vi "BuildSysexMsgCapabilityQuery.vi"(8 "error in":errorcluster) -> (0 "error out":errorcluster, 2 "GetCapabilitiesMessage":u8[](array[numeric]) format="%x", 4 "ReplyFirstByte":T1=224 items=["ANALOG_IO_MESSAGE"=224, "DIGITAL_IO_MESSAGE"=144, "REPORT_ANALOG_PIN"=192, "REPORT_DIGITAL_PORT"=208, "START_SYSEX"=240, "END_SYSEX"=247, "SET_PIN_MODE"=244, "SET_DIGITAL_PIN_VALUE"=245, "PROTOCOL_VERSION"=249, "SYSTEM_RESET"=255, "SYSEX.EXTENDED_ID"=0, "SYSEX.RESERVED_USER_COMMANDs"=1, "SYSEX.ANALOG_MAPPING_QUERY"=105, "SYSEX.ANALOG_MAPPING_RESPONSE"=106, "SYSEX.CAPABILITY_QUERY"=107, "SYSEX.CAPABILITY_RESPONSE"=108, "SYSEX.PIN_STATE_QUERY"=109, "SYSEX.PIN_STATE_RESPONSE"=110, "SYSEX.REPORT_FIRMWARE"=121, "SYSEX.EXTENDED_ANALOG"=111, "SYSEX.STRING_DATA"=113, "SYSEX.REALTIME"=127, "SYSEX.NON_REALTIME"=126, "SYSEX.SAMPLING_INTERVAL"=122, "FEATURES.SYSEX.I2C_READ_WRITE"=118, "FEATURES.SYSEX.I2C_REPLY"=119, "FEATURES.SYSEX.I2C_CONFIG"=120], 6 "ReplyLength":i32=-1)   [LabVIEW 2020, in "FirmataClient.lvlib"]
doc: "Builds the message according to the Firmata Protocol Requirements. \n- https://github.com/firmata/protocol\n- https://github.com/firmata/protocol/blob/master/protocol.md"
uses:
  Controls/FirmataProtocolConstants.ctl
  FirmataClient.lvlib
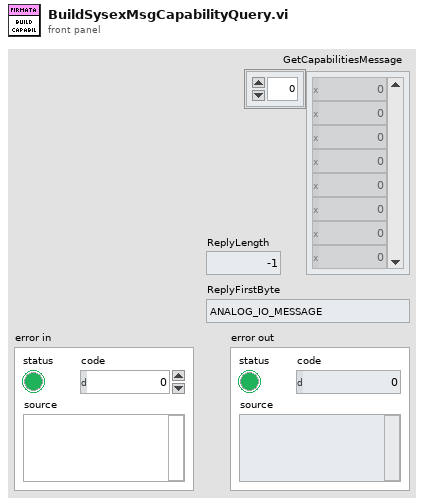
[diagram p1: front panel]
types:
  T1 = typedef "FirmataClient.lvlib/FirmataProtocolConstants.ctl" = u16
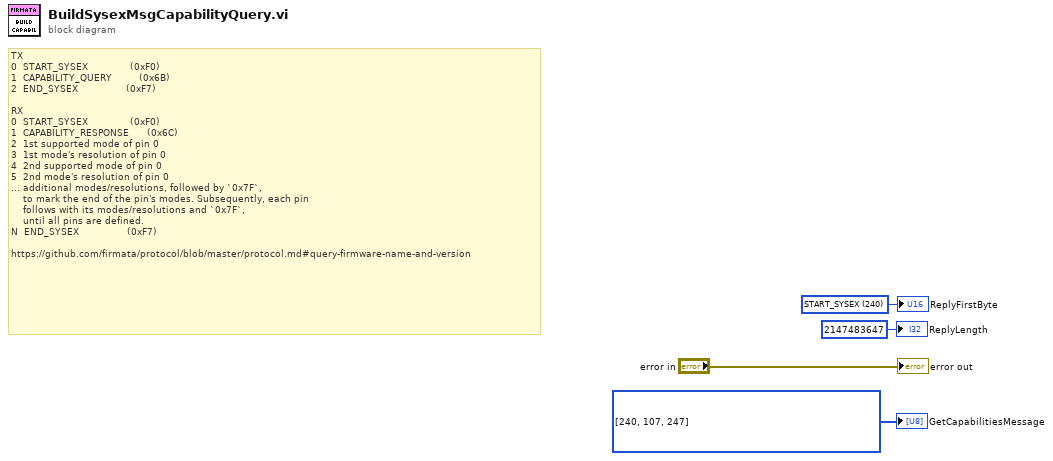
[diagram p0: block diagram]
diagram:
  w1 = T1 240 items=["ANALOG_IO_MESSAGE"=224, "DIGITAL_IO_MESSAGE"=144, "REPORT_ANALOG_PIN"=192, "REPORT_DIGITAL_PORT"=208, "START_SYSEX"=240, "END_SYSEX"=247, "SET_PIN_MODE"=244, "SET_DIGITAL_PIN_VALUE"=245, "PROTOCOL_VERSION"=249, "SYSTEM_RESET"=255, "SYSEX.EXTENDED_ID"=0, "SYSEX.RESERVED_USER_COMMANDs"=1, "SYSEX.ANALOG_MAPPING_QUERY"=105, "SYSEX.ANALOG_MAPPING_RESPONSE"=106, "SYSEX.CAPABILITY_QUERY"=107, "SYSEX.CAPABILITY_RESPONSE"=108, "SYSEX.PIN_STATE_QUERY"=109, "SYSEX.PIN_STATE_RESPONSE"=110, "SYSEX.REPORT_FIRMWARE"=121, "SYSEX.EXTENDED_ANALOG"=111, "SYSEX.STRING_DATA"=113, "SYSEX.REALTIME"=127, "SYSEX.NON_REALTIME"=126, "SYSEX.SAMPLING_INTERVAL"=122, "FEATURES.SYSEX.I2C_READ_WRITE"=118, "FEATURES.SYSEX.I2C_REPLY"=119, "FEATURES.SYSEX.I2C_CONFIG"=120] ("ReplyFirstByte")
  w3 = T1[] [240, 107, 247] items=["ANALOG_IO_MESSAGE"=224, "DIGITAL_IO_MESSAGE"=144, "REPORT_ANALOG_PIN"=192, "REPORT_DIGITAL_PORT"=208, "START_SYSEX"=240, "END_SYSEX"=247, "SET_PIN_MODE"=244, "SET_DIGITAL_PIN_VALUE"=245, "PROTOCOL_VERSION"=249, "SYSTEM_RESET"=255, "SYSEX.EXTENDED_ID"=0, "SYSEX.RESERVED_USER_COMMANDs"=1, "SYSEX.ANALOG_MAPPING_QUERY"=105, "SYSEX.ANALOG_MAPPING_RESPONSE"=106, "SYSEX.CAPABILITY_QUERY"=107, "SYSEX.CAPABILITY_RESPONSE"=108, "SYSEX.PIN_STATE_QUERY"=109, "SYSEX.PIN_STATE_RESPONSE"=110, "SYSEX.REPORT_FIRMWARE"=121, "SYSEX.EXTENDED_ANALOG"=111, "SYSEX.STRING_DATA"=113, "SYSEX.REALTIME"=127, "SYSEX.NON_REALTIME"=126, "SYSEX.SAMPLING_INTERVAL"=122, "FEATURES.SYSEX.I2C_READ_WRITE"=118, "FEATURES.SYSEX.I2C_REPLY"=119, "FEATURES.SYSEX.I2C_CONFIG"=120]
  # "TX\n0  START_SYSEX              (0xF0)\n1  CAPABILITY_QUERY         (0x6B)\n2  END_SYSEX                (0xF7)\n\nRX\n0  START_SYSEX              (0xF0)\n1  CAPABILITY_RESPONSE      (0x6C)\n2  1st supported mode of pin 0\n3  1st mode's resolution of pin 0\n4  2nd supported mode of pin 0\n5  2nd mode's resolution of pin 0\n... additional modes/resolutions, followed by `0x7F`,\n    to mark the end of the pin's modes. Subsequently, each pin\n    follows with its modes/resolutions and `0x7F`,\n    until all pins are defined.\nN  END_SYSEX                (0xF7)\n\nhttps://github.com/firmata/protocol/blob/master/protocol.md#query-firmware-name-and-version"
  "error out" <- "error in"
  "GetCapabilitiesMessage" <- w3
  "ReplyFirstByte" <- w1
  "ReplyLength" <- 2147483647 ("ReplyLength")
